vi "Simulation - Wall Detection.vi"() -> ()   [LabVIEW 2013]
doc: "This VI starts and stops the environment simulator and serves as the master VI for your simulation code. Open and run this VI to display the environment simulator, or open the block diagram to view or modify simulation code."
uses:
  <vilib>/robotics/Simulator/Engine/ctl/DeviceID.ctl
  <instrlib>/DC Motor Controller/HAIOL/DC Motor Controller.lvclass
  <instrlib>/Hokuyo URG Series/HAIOL/Hokuyo URG Series.lvclass
  <vilib>/robotics/Simulator/NI_Robotics_Simulator.lvlib
  <instrlib>/DC Motor Controller/HAIOL/Simulator/DC Motor Controller Simulator.lvclass
  <instrlib>/Hokuyo URG Series/HAIOL/Simulator/Hokuyo URG Series Simulator.lvclass
panel:
  out "XY Graph":cluster{"X":dbl, "Y":dbl}[](graph)
  in  "Speed":dbl(slide) scale=0.0..20.0
  in  "Direction":dbl
  in  "stop":bool
  out "3D Picture":refnum<vi>(3d-picture)
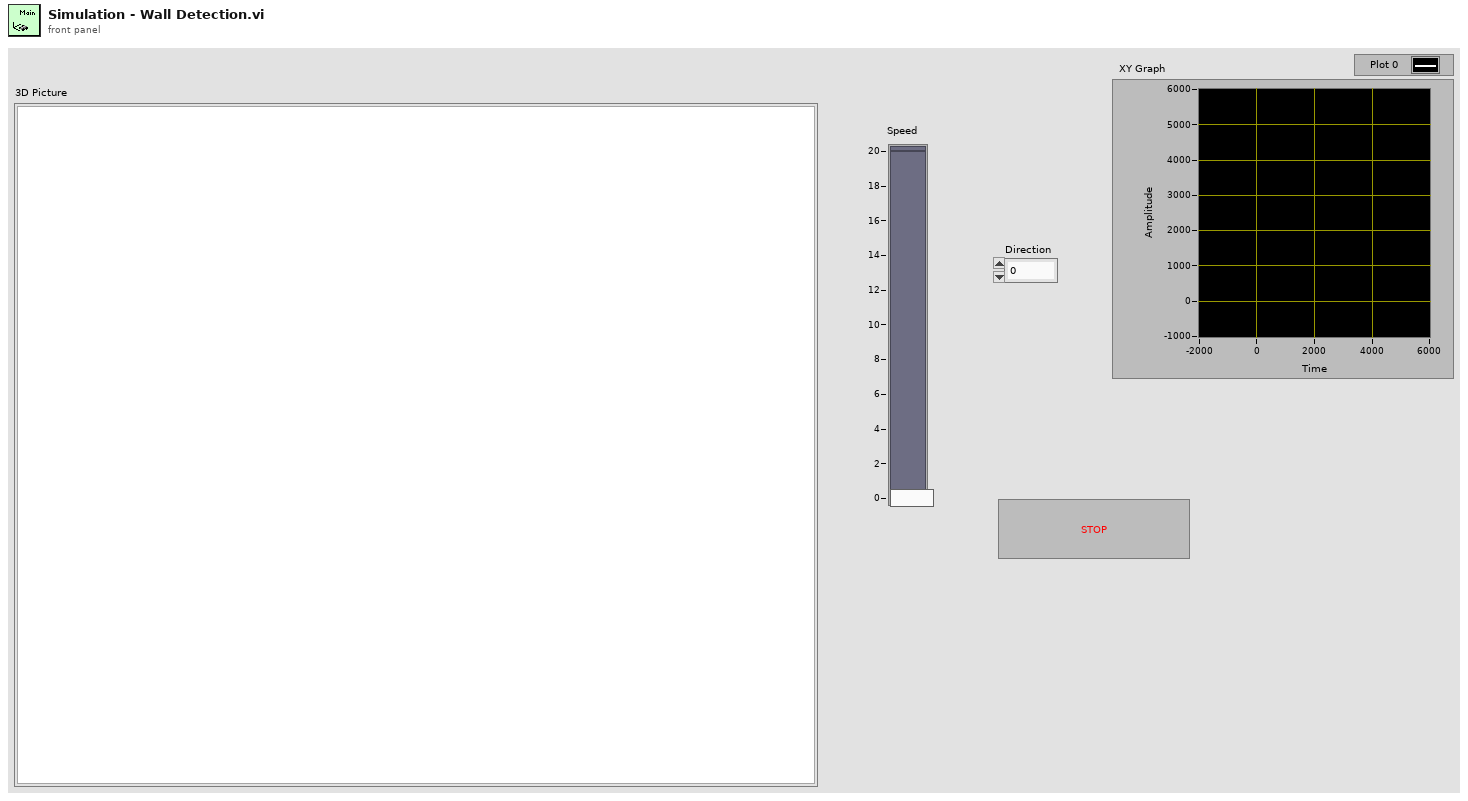
[diagram p1: front panel]
types:
  T1 = typedef "NI_Robotics_Simulator.lvlib/DeviceID.ctl" = cluster{"robot ID":string, "sensor/actuator ID":string}
  T2 = cluster{"current angle":dbl, "current count":i32}
  T3 = cluster{"DC Motor Controller out":refnum<class "DC Motor Controller.lvclass">, "DC Motor Controller out":refnum<class "DC Motor Controller.lvclass">, "DC Motor Controller out":refnum<class "DC Motor Controller.lvclass">}
  T4 = cluster{"current count":i32, "current angle":dbl}
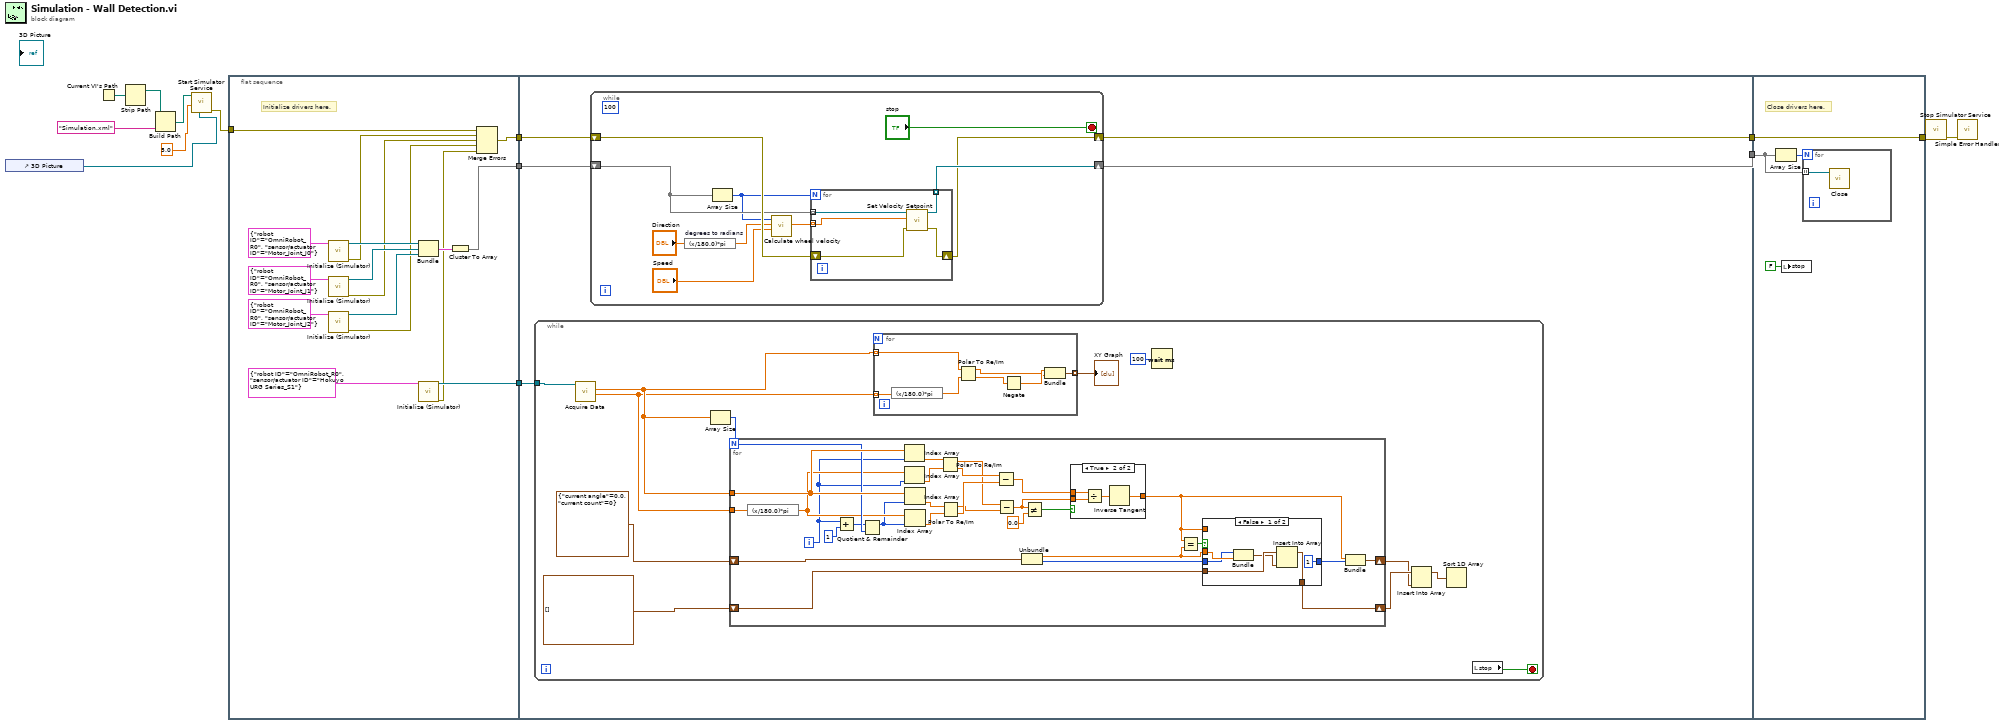
[diagram p0: block diagram]
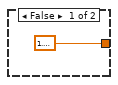
[diagram p2: hidden frame]
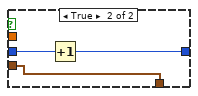
[diagram p3: hidden frame]
diagram:
  n1 = control-ref of="3D Picture"() -> (w2:refnum<vi>)
  n2 = Current VI's Path() -> (path=w13:path)
  n3 = Strip Path(path=w13) -> (stripped path=w12:path)  [unwired: 1 out]
  n4 = Build Path(base path=w12, name or relative path="Simulation.xml" ("manifest filename")) -> (appended path=w5:path)
  n5 = call <vilib>:"Start Simulator Service.vi"("3D picture refnum"=w2, "step size (ms)"=5.0 ("stepsize(ms)"), "manifest file"=w5) -> ("error out"=w3:errorcluster)  [unwired: 8 in]
  n6 = flat-sequence {
    tunnel: w3 -> [w26]
    tunnel: [w25] -> w10
    tunnel: [w28] -> w7
    tunnel: [w16] -> w1
    tunnel: w10 -> [w34]
    tunnel: [w35] -> w9
    tunnel: w7 -> [w33]
    tunnel: [w32] -> w6
    tunnel: w1 -> [w31]
    tunnel: [w116] -> w14
    tunnel: w9 -> [w116]
    tunnel: w6 -> [w114]
    frame #0 {
      # "Initialize drivers here."
      n7 = call <instrlib>:"Initialize (Simulator).vi"("Device ID"=T1 {"robot ID"="OmniRobot_R0", "sensor/actuator ID"="Motor_Joint_J0"}) -> ("error out"=w24:errorcluster, "DC Motor Controller out"=w29:refnum<class "DC Motor Controller.lvclass">)  [unwired: 9 in]
      n8 = call <instrlib>:"Initialize (Simulator).vi"("Device ID"=T1 {"robot ID"="OmniRobot_R0", "sensor/actuator ID"="Motor_Joint_J1"}) -> ("error out"=w20:errorcluster, "DC Motor Controller out"=w23:refnum<class "DC Motor Controller.lvclass">)  [unwired: 9 in]
      n9 = call <instrlib>:"Initialize (Simulator).vi"("Device ID"=T1 {"robot ID"="OmniRobot_R0", "sensor/actuator ID"="Motor_Joint_J2"}) -> ("error out"=w21:errorcluster, "DC Motor Controller out"=w22:refnum<class "DC Motor Controller.lvclass">)  [unwired: 9 in]
      n10 = Bundle("DC Motor Controller out"=w29, "DC Motor Controller out"=w23, "DC Motor Controller out"=w22) -> (w27:T3)  [unwired: 1 in]
      n11 = call <instrlib>:"Initialize (Simulator).vi"("Device ID"=T1 {"robot ID"="OmniRobot_R0", "sensor/actuator ID"="Hokuyo URG Series_S1"}) -> ("Hokuyo URG Series out"=w16:refnum<class "Hokuyo URG Series.lvclass">, "error out"=w15:errorcluster)  [unwired: 13 in]
      n12 = Cluster To Array(cluster=w27) -> (array=w28:refnum<class "DC Motor Controller.lvclass">[])
      n13 = Merge Errors(w26, w24, w20, w21, w15) -> (w25:errorcluster)
    }
    frame #1 {
      n14 = while {
        tunnel: w31 -> [w47]
        stop <- w42 stop-if-true
        n15 = call-dynamic "Acquire Data.vi"("Hokuyo URG Series in"=w47) -> ("Direction"=w37:dbl[], "Magnitude"=w38:dbl[])  [unwired: 7 in, 2 out]
        n16 = Array Size(array=w38) -> (size(s)=w45:i32)
        n17 = for {
          N: w45 -> [w73]
          tunnel: w38 -> [w83]
          tunnel: w37 -> [w60]
          shift-right: [w65] -> w40
          shift-left: cluster{"angle":dbl, "count":i32}[] [] -> [w67]
          shift-right: [w71] -> w39
          shift-left: T2 {"current angle"=0.0, "current count"=0} -> [w72]
          i -> [w56]
          n18 = expression code="(x/180.0)*pi" ("degrees to radians")(w60) -> (w59:dbl[])
          n19 = Add(x=w56, y=1) -> (x+y=w58:i32)
          n20 = Quotient & Remainder(x=w58, y=w73) -> (x-y*floor(x/y)=w55:i32)  [unwired: 1 out]
          n21 = Index Array(array=w83, index=w56) -> (element=w81:dbl)
          n22 = Index Array(array=w59, index=w56) -> (element=w82:dbl)
          n23 = Index Array(array=w83, index=w55) -> (element=w80:dbl)
          n24 = Index Array(array=w59, index=w55) -> (element=w79:dbl)
          n25 = Polar To Re/Im(2:w82, 3:w81) -> (0:w77:dbl, 1:w76:dbl)
          n26 = Polar To Re/Im(2:w79, 3:w80) -> (0:w78:dbl, 1:w75:dbl)
          n27 = Subtract(x=w77, y=w78) -> (x-y=w74:dbl)
          n28 = Subtract(x=w76, y=w75) -> (x-y=w63:dbl)
          n29 = Unbundle(w72) -> ("current angle"=w66:dbl, "current count"=w69:i32)
          n30 = Not Equal?(x=w63, y=0.0) -> (x != y?=w61:bool)
          n31 = case shown="True" w61 {
            tunnel: w74 -> [_ w85]
            tunnel: w63 -> [_ w87]
            tunnel: [1.5707963267948966 w86] -> w64
            frame False {
            }
            frame True {
              n32 = Divide(x=w85, y=w87) -> (x/y=w88:dbl)
              n33 = Inverse Tangent(1:w88) -> (0:w86:dbl)
            }
          }
          n34 = Equal?(x=w64, y=w66) -> (x = y?=w70:bool)
          n35 = case shown="False" w70 {
            tunnel: w69 -> [w90 w97]
            tunnel: [1 w96] -> w68
            tunnel: w67 -> [w94 w95]
            tunnel: w66 -> [w91 _]
            tunnel: [w92 w95] -> w65
            tunnel: w64 -> [_ _]
            frame False {
              n36 = Bundle("current count"=w90, "current angle"=w91) -> (w93:T4)  [unwired: 1 in]
              n37 = Insert Into Array(array=w94, new element=w93) -> (w92:cluster{"angle":dbl, "count":i32}[])  [unwired: 1 in]
            }
            frame True {
              n38 = Increment(x=w97) -> (x+1=w96:i32)
            }
          }
          n39 = Bundle(w64, w68) -> (w71:cluster{dbl, i32})  [unwired: 1 in]
        }
        n40 = for {
          tunnel: w38 -> [w52] mode=indexing
          tunnel: w37 -> [w54] mode=indexing
          tunnel: [w51] -> w36 mode=indexing
          n41 = expression code="(x/180.0)*pi" ("degrees to radians")(w54) -> (w53:dbl)
          n42 = Polar To Re/Im(2:w53, 3:w52) -> (0:w49:dbl, 1:w48:dbl)
          n43 = Negate(x=w49) -> (-x=w50:dbl)
          n44 = Bundle(w50, w48) -> (w51:cluster{dbl, dbl})  [unwired: 1 in]
        }
        "XY Graph" <- w36
        n45 = Wait (ms)(milliseconds to wait=u32 100) -> ()  [unwired: 1 out]
        n46 = Insert Into Array(array=w40, new element=w39) -> (w41:cluster{"angle":dbl, "count":i32}[])  [unwired: 1 in]
        n47 = Sort 1D Array(array=w41) -> ()  [unwired: 1 out]
        n48 = local read "stop"() -> (w42:bool)
      }
      n49 = while {
        shift-right: [w104] -> w35
        shift-left: w34 -> [w107]
        shift-right: [w105] -> w32
        shift-left: w33 -> [w106]
        stop <- "stop" stop-if-true
        (unwired) 100
        n50 = expression code="(x/180.0)*pi" "degrees to radians"("Direction") -> (w100:dbl)
        n51 = Array Size(array=w106) -> (size(s)=w103:i32)
        n52 = call "Calculate wheel velocity.vi"("Speed"="Speed", "Direction (radians)"=w100, "Number of Wheels"=w103) -> ("Wheel speeds"=w102:dbl[])  [unwired: 8 in]
        n53 = for {
          N: w103 -> [_]
          tunnel: w106 -> [w112] mode=indexing
          tunnel: w102 -> [w108] mode=indexing
          shift-right: [w110] -> w104
          shift-left: w107 -> [w111]
          tunnel: [w109] -> w105 mode=indexing
          n54 = call-dynamic "Set Velocity Setpoint.vi"("error in (no error)"=w111, "CCW Velocity (0 rad/s)"=w108, "DC Motor Controller in"=w112) -> ("error out"=w110:errorcluster, "DC Motor Controller out"=w109:refnum<class "DC Motor Controller.lvclass">)  [unwired: 7 in]
        }
      }
    }
    frame #2 {
      # "Close drivers here."
      n55 = Array Size(array=w114) -> (size(s)=w115:i32)
      n56 = local write "stop"(FALSE ("stop")) -> ()
      n57 = for {
        N: w115 -> [_]
        tunnel: w114 -> [w117] mode=indexing
        n58 = call-dynamic "Close.vi"("DC Motor Controller in"=w117) -> ()  [unwired: 10 in, 1 out]
      }
    }
  }
  n59 = call <vilib>:"Stop Simulator Service.vi"("error in (no error)"=w14) -> ("error out"=w11:errorcluster)  [unwired: 10 in]
  n60 = call <vilib>:"Simple Error Handler.vi"("error in (no error)"=w11) -> ()  [unwired: 4 in, 5 out]
